vi "Run Tests.vi"() -> ()   [LabVIEW 2019, in "Test Redis Client for LabVIEW.lvlib"]
uses:
  Test Redis Client for LabVIEW.lvlib
  <vilib>/Utility/miscctls.llb/LVRowAndColumnTypeDef.ctl
  <vilib>/Analysis/baseanly.llb/Mean (DBL).vi
  <vilib>/regexp/Match Regular Expression.xnode
  <vilib>/ptbypt/NI_PtbyPt.lvlib
  <vilib>/gmath/NI_Gmath.lvlib
  <vilib>/Analysis/NI_AALBase.lvlib
  Test Redis Client/Test Redis Client.lvclass
panel:
  in  "min iters":i32=10
  in  "max iters":i32=100
  out "current test":string
  out "Test Results":string[][](table)
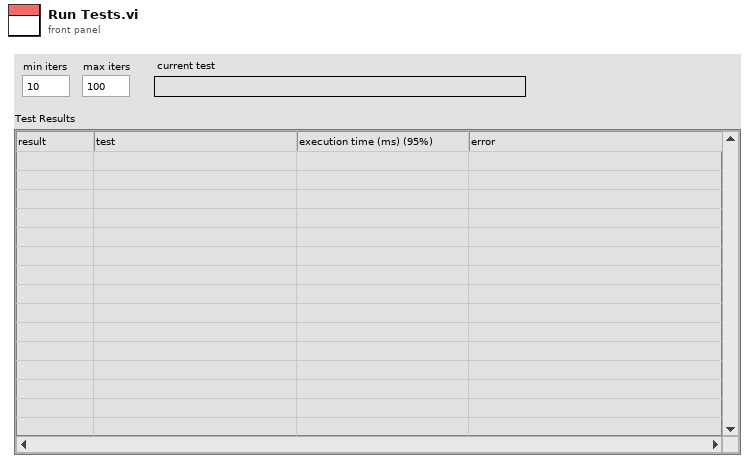
[diagram p1: front panel]
types:
  T1 = typedef "LVRowAndColumnTypeDef.ctl" = cluster{"Row":i32, "Column":i32}
  T2 = cluster{string, "pass?":bool, "error IO":errorcluster, "mean":dbl, "confidence interval":cluster{"low":dbl, "high":dbl}}
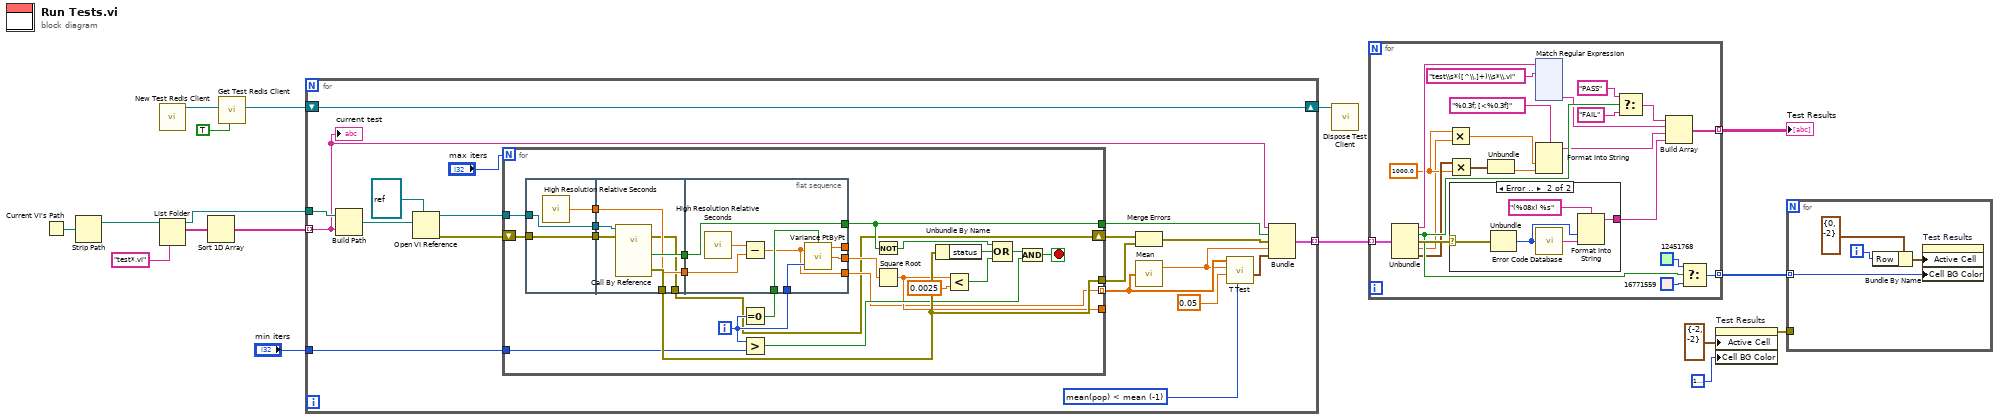
[diagram p0: block diagram]
diagram:
  n1 = Current VI's Path() -> (path=w17:path)
  n2 = Strip Path(path=w17) -> (stripped path=w16:path)  [unwired: 1 out]
  n3 = call "New Test Redis Client.vi"() -> ("Test Redis Client out"=w3:refnum<class "Test Redis Client.lvclass">)  [unwired: 8 in, 3 out]
  n4 = List Folder(path=w16, pattern="test*.vi") -> (path out=w12:path, filenames=w14:string[])  [unwired: 2 in, 2 out]
  n5 = Sort 1D Array(array=w14) -> (sorted array=w13:string[])
  n6 = call "Get Test Redis Client.vi"("(T) Set / (F) Get"=TRUE, "Test Client In"=w3) -> ("Test Client Out"=w2:refnum<class "Test Redis Client.lvclass">)  [unwired: 9 in]
  n7 = for {
    tunnel: w13 -> [w26] mode=indexing
    tunnel: w12 -> [w35]
    tunnel: [w27] -> w11 mode=indexing
    tunnel: "min iters" -> [w19]
    shift-right: [w18] -> w1
    shift-left: w2 -> [w18]
    w22 = -1 items=["mean(pop) != mean"=0, "mean(pop) > mean"=1, "mean(pop) < mean"=-1] ("alternative hypothesis")
    n8 = Build Path(base path=w35, name or relative path=w26) -> (appended path=w34:path)
    n9 = Open VI Reference(type specifier VI Refnum (for type only)=refnum<vi> refnum, vi path=w34) -> (vi reference=w33:refnum<vi>, error out=w32:errorcluster)  [unwired: 4 in]
    n10 = for {
      N: "max iters" -> [_]
      tunnel: w33 -> [w59]
      tunnel: [w57] -> w30
      tunnel: [w55] -> w29
      shift-right: [w39] -> w31
      shift-left: w32 -> [w58]
      tunnel: [w42] -> _
      tunnel: [w41] -> w24 mode=indexing
      tunnel: w19 -> [w40]
      i -> [w46]
      stop <- w45 stop-if-true
      n11 = flat-sequence {
        tunnel: w58 -> [w61]
        tunnel: w59 -> [w62]
        tunnel: [w62] -> w52
        tunnel: [w61] -> w51
        tunnel: [w60] -> w50
        tunnel: [w66] -> w57
        tunnel: [w65] -> w38
        tunnel: w52 -> [w68]
        tunnel: w51 -> [w67]
        tunnel: w50 -> [w64]
        tunnel: [w64] -> w37
        tunnel: [w63] -> w39
        tunnel: [w76] -> w55
        tunnel: w38 -> [w76]
        tunnel: w37 -> [w74]
        tunnel: w49 -> [w73]
        tunnel: w46 -> [w72]
        tunnel: [w71] -> _
        tunnel: [w70] -> w43
        tunnel: [w69] -> w41
        frame #0 {
          n12 = call <vilib>:"High Resolution Relative Seconds.vi"() -> ("relative seconds"=w60:dbl)
        }
        frame #1 {
          n13 = call-by-ref "?"(reference=w68, error in=w67) -> (error out=w63:errorcluster, 0:"error out"=w66:errorcluster, "pass?"=w65:bool)  [unwired: 10 in, 1 out]
        }
        frame #2 {
          n14 = call <vilib>:"High Resolution Relative Seconds.vi"() -> ("relative seconds"=w75:dbl)
          n15 = Subtract(x=w75, y=w74) -> (x-y=w69:dbl)
          n16 = call <vilib>:"Variance PtByPt.vi"("x"=w69, "sample length"=w72, "initialize"=w73) -> ("mean"=w71:dbl, "variance"=w70:dbl)  [unwired: 1 out]
        }
      }
      n17 = Equal To 0?(x=w46) -> (x = 0?=w49:bool)
      n18 = Greater?(x=w46, y=w40) -> (0:w44:bool)
      n19 = Not(x=w55) -> (.not. x?=w54:bool)
      n20 = Square Root(x=w43) -> (sqrt(x)=w42:dbl)
      n21 = Unbundle By Name(w57) -> ("status"=w56:bool)
      n22 = Less?(x=w42, y=0.0025) -> (x < y?=w47:bool)
      n23 = Compound Arithmetic op=OR(w54, w56, w47) -> (w53:bool)
      n24 = Compound Arithmetic op=AND(w53, w44) -> (w45:bool)
    }
    n25 = Merge Errors(w31, w30) -> (w28:errorcluster)
    n26 = call-poly <vilib>:"Mean.vi"("X"=w24) -> ("mean"=w20:dbl)  [unwired: 1 out]
    n27 = call <vilib>:"T Test.vi"("alternative hypothesis"=w22, "significance level"=0.05, "mean"=w20, "sample set"=w24) -> ("confidence interval"=w21:cluster{"low":dbl, "high":dbl})  [unwired: 3 in, 4 out]
    n28 = Bundle(w26, "pass?"=w29, "error IO"=w28, "mean"=w20, "confidence interval"=w21) -> (w27:T2)  [unwired: 1 in]
    "current test" <- w26
  }
  n29 = call "Dispose Test Client.vi"("Test Redis Client in"=w1) -> ()  [unwired: 10 in, 1 out]
  n30 = for {
    tunnel: w11 -> [w98] mode=indexing
    tunnel: [w91] -> w10 mode=indexing
    tunnel: [w89] -> w9 mode=indexing
    w79 = 1000.0 ("y")
    n31 = Unbundle(w98) -> (w87:string, "pass?"=w94:bool, "error IO"=w95:errorcluster, "mean"=w78:dbl, "confidence interval"=w82:cluster{"low":dbl, "high":dbl})
    n32 = Multiply(x=w79, y=w78) -> (x*y=w77:dbl)
    n33 = Multiply(x=w82, y=w79) -> (x*y=w81:cluster{"low":dbl, "high":dbl})
    n34 = case shown="Error .." w95 {
      selector: w95 -> [_ w217]
      tunnel: [_ w218] -> w85
      frame No Error {
      }
      frame Error {
        n35 = Unbundle(w217) -> ("code"=w216:i32)  [unwired: 2 out]
        n36 = call <vilib>:"Error Code Database.vi"("Error Code"=w216) -> ("Error Text"=w215:string)
        n37 = Format Into String(format string="(%08x) %s", w216, w215) -> (resulting string=w218:string)  [unwired: 2 in, 1 out]
      }
    }
    n38 = Unbundle(w81) -> ("high"=w80:dbl)  [unwired: 1 out]
    n39 = xnode "Match Regular Expression"("input string"=w87, "regular expression"="test\\s*([^\\.]+)\\s*\\.vi") -> ("submatch 1"=w86:string)  [unwired: 4 in, 5 out]
    n40 = Format Into String(format string="%0.3f; [<%0.3f]", w77, w80) -> (resulting string=w83:string)  [unwired: 2 in, 1 out]
    n41 = Select(t="PASS", s=w94, f="FAIL") -> (s? t:f=w90:string)
    n42 = Build Array(w90, w86, w83, w85) -> (w91:string[])
    n43 = Select(t=u32 12451768, s=w94, f=u32 16771559) -> (s? t:f=w89:u32)
  }
  "Test Results" <- w10
  n44 = property on="Test Results" class="Tbl (strict)"("Active Cell"=T1 {"Row"=-2, "Column"=-2} ("Active Cell:Active Cell"), "Cell BG Color"=u32 16777225 ("Active Cell:Cell Background Color")) -> (error out=w8:errorcluster)  [unwired: 2 in, 1 out]
  n45 = for {
    tunnel: w9 -> [w220] mode=indexing
    tunnel: w8 -> [_]
    i -> [w222]
    n46 = Bundle By Name(cluster=T1 {"Row"=0, "Column"=-2} ("Active Cell:Active Cell"), "Row"=w222) -> (w221:T1)
    n47 = property on="Test Results" class="Tbl (strict)"("Active Cell"=w221, "Cell BG Color"=w220) -> ()  [unwired: 2 in, 2 out]
  }
